vi "Get Speed.vi"(8 "error in (no error)":errorcluster, 11 "FINE SIM Motion Axis":refnum<class "FINE SIM Motion Axis.lvclass">) -> (0 "error out":errorcluster, 2 "Axis Speed":dbl, 3 "FINE SIM Motion Axis":refnum<class "FINE SIM Motion Axis.lvclass">)   [LabVIEW 2022 SP3, in "FINE SIM Motion Axis.lvclass"]
uses:
  FINE SIM Motion Axis.lvclass
  FINE SIM Motion Axis.lvclass/FINE SIM Motion Axis.ctl
  Accessors/Read Sim Axis Data.vi
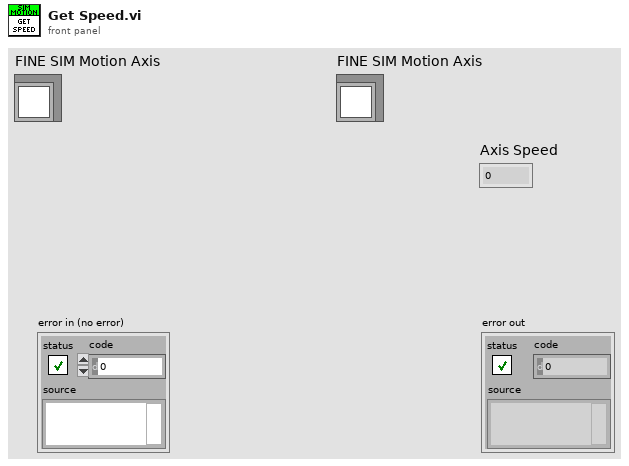
[diagram p1: front panel]
types:
  T1 = typedef "FINE SIM Motion Axis.lvclass/Axis Data.ctl" = cluster{"Axis Parameters":T2, "Time Stamp":timestamp, "Settings":T4}
  T2 = typedef "FINE SIM Motion Axis.lvclass/Axis Parameters.ctl" = cluster{"Moving":bool, "Homed":bool, "Desired Position":dbl, "Current Positon":dbl, "Current Speed":dbl, "Home Status":T3}
  T3 = typedef "FINE SIM Motion Axis.lvclass/Homing Status.ctl" = enum16{"Idle", "Inital Home Motion", "Final Home Motion", "Done Homing"}
  T4 = typedef "FINE SIM Motion Axis.lvclass/Settings.ctl" = cluster{"Axis Name":string, "Axis Settings":T5}
  T5 = typedef "FINE SIM Motion Axis.lvclass/Axis Settings.ctl" = cluster{"Speed":dbl, "Acceleration":dbl}
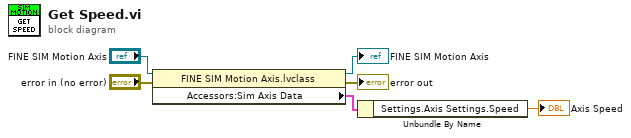
[diagram p0: block diagram]
diagram:
  n1 = property class="FINE SIM Motion Axis.lvclass"(reference="FINE SIM Motion Axis", error in="error in (no error)") -> (reference out=→"FINE SIM Motion Axis":refnum<class "FINE SIM Motion Axis.lvclass">, error out=→"error out":errorcluster, "Accessors:Sim Axis Data"=w6:T1)
  n2 = Unbundle By Name(w6) -> ("Settings.Axis Settings.Speed"=→"Axis Speed":dbl)
